vi "点堆模拟机物理参数设置.vi"() -> ()   [LabVIEW 2020]
panel:
  in  "其他说明":string
  in  "文字说明":string
  in  "Lamda 6":sgl
  in  "Lamda 5":sgl
  in  "Lamda 4":sgl
  in  "Lamda 3":sgl
  in  "Lamda 2":sgl
  in  "Beta 6":sgl
  in  "Beta 5":sgl
  in  "Beta 4":sgl
  in  "Beta 3":sgl
  in  "Beta 2":sgl
  in  "取消修改":bool caption="Cancel Button"
  in  "保存修改":bool
  in  "Lamda 1":sgl
  in  "Beta 1":sgl
  in  "源强":sgl
  in  "中子寿命":sgl
  # "点堆模拟机物理参数设置"
  # "（参数对应堆型等）"
  # "（修改日期时间等）"
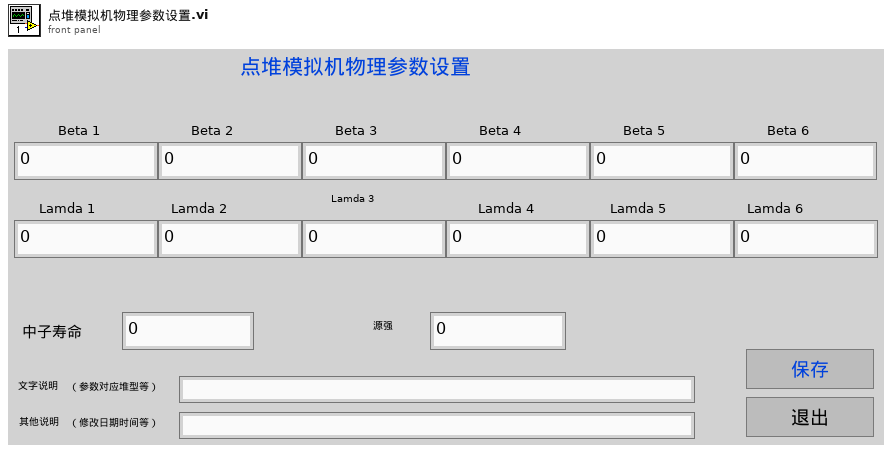
[diagram p1: front panel]
types:
  T1 = enum16{"open", "replace", "create", "open or create", "replace or create", "replace or create with confirmation"}
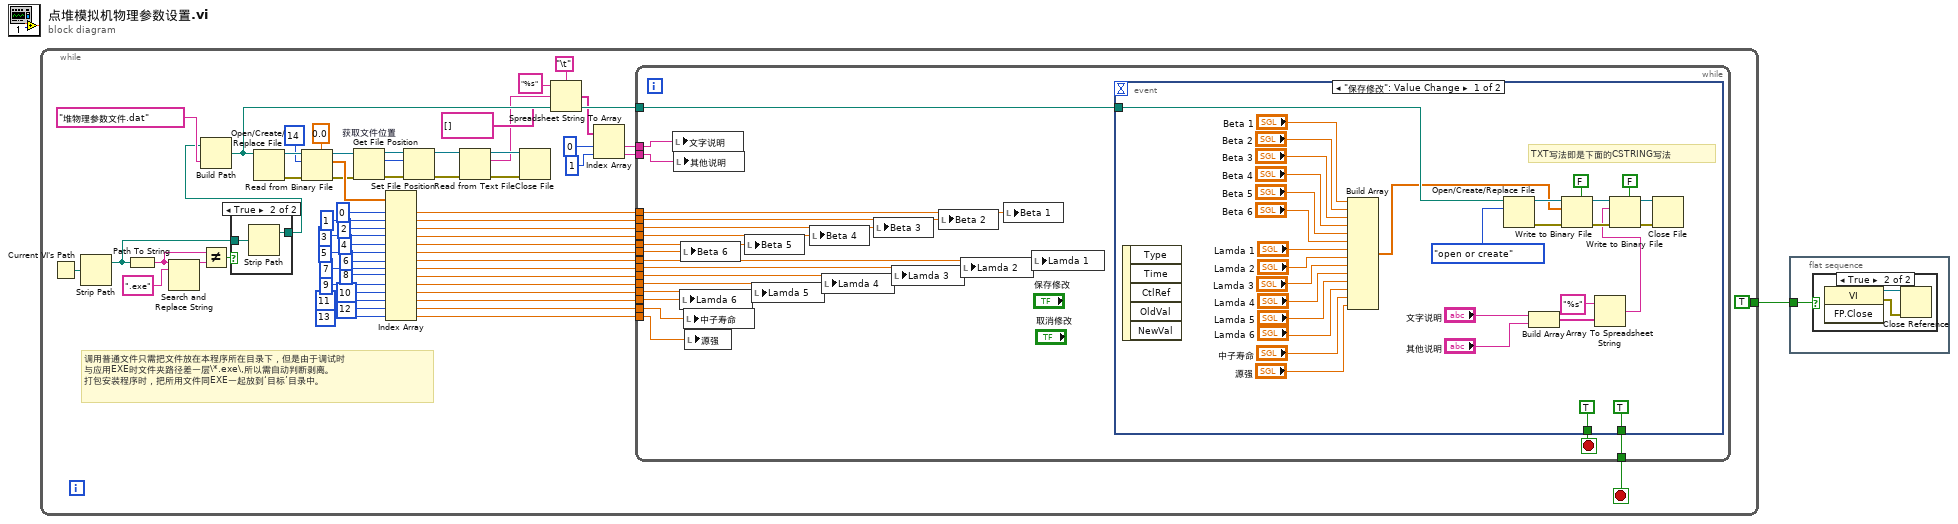
[diagram p0: block diagram]
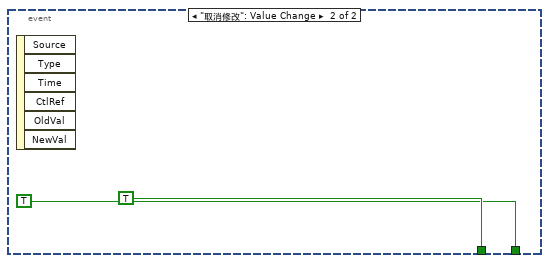
[diagram p4: hidden frame]
diagram:
  n1 = while {
    tunnel: [TRUE] -> w1
    stop <- w38 stop-if-true
    # "调用普通文件只需把文件放在本程序所在目录下，但是由于调试时\n与应用EXE时文件夹路径差一层\\*.exe\\,所以需自动判断剥离。\n打包安装程序时，把所用文件同EXE一起放到‘目标’目录中。"
    n2 = Current VI's Path() -> (path=w9:path)
    n3 = Strip Path(path=w9) -> (stripped path=w4:path)  [unwired: 1 out]
    n4 = Path To String(path=w4) -> (string=w6:string)
    n5 = Search and Replace String(input string=w6, search string=".exe" ("搜索字符串")) -> (result string=w7:string)  [unwired: 6 in, 3 out]
    n6 = Not Equal?(x=w6, y=w7) -> (x != y?=w5:bool)
    n7 = case shown="True" w5 {
      tunnel: w4 -> [w64 w66]
      tunnel: [w64 w65] -> w3
      frame False {
      }
      frame True {
        n8 = Strip Path(path=w66) -> (stripped path=w65:path)  [unwired: 1 out]
      }
    }
    n9 = Build Path(base path=w3, name or relative path="堆物理参数文件.dat") -> (appended path=w36:path)
    n10 = Open/Create/Replace File(file path (use dialog)=w36) -> (refnum out=w49:refnum<file>, error out=w48:errorcluster)  [unwired: 5 in, 1 out]
    n11 = Read from Binary File(5:sgl 0.0 ("byte stream type"), 8:w48, 10:14 ("count"), 11:w49) -> (0:w34:errorcluster, 2:w45:sgl[], 3:w35:refnum<file>)  [unwired: 2 in, 1 out]
    n12 = Get File Position "获取文件位置"(4:w34, 7:w35) -> (0:w43:errorcluster, 2:w19:i64, 3:w44:refnum<file>)
    n13 = Index Array(array=w45, index #1=0, index #2=1, index #3=2, index #4=3, index #5=4, index #6=5, index #7=6, index #8=7, index #9=8, index #10=9, index #11=10, index #12=11, index #13=12, index #14=13) -> (element #1=w33:sgl, element #2=w32:sgl, element #3=w31:sgl, element #4=w30:sgl, element #5=w29:sgl, element #6=w28:sgl, element #7=w27:sgl, element #8=w26:sgl, element #9=w25:sgl, element #10=w24:sgl, element #11=w23:sgl, element #12=w22:sgl, element #13=w21:sgl, element #14=w20:sgl)
    n14 = Set File Position(offset (in bytes) (0)=w19, refnum=w44, error in=w43) -> (refnum out=w18:refnum<file>, error out=w17:errorcluster)  [unwired: 1 in]
    n15 = Read from Text File(file (use dialog)=w18, error in=w17) -> (refnum out=w16:refnum<file>, text=w11:string, error out=w15:errorcluster)  [unwired: 1 in, 2 out]
    n16 = Close File(refnum=w16, error in=w15) -> ()  [unwired: 2 out]
    n17 = Spreadsheet String To Array(delimiter (Tab)="\t", format string="%s", spreadsheet string=w11, array type (2D Dbl)=string[] [] ("添加的数组")) -> (array=w10:string[])
    n18 = Index Array(array=w10, index #1=0 ("index"), index #2=1 ("index")) -> (element #1=w40:string, element #2=w39:string)
    n19 = while {
      tunnel: w33 -> [w85]
      tunnel: w32 -> [w84]
      tunnel: w31 -> [w83]
      tunnel: w30 -> [w82]
      tunnel: w29 -> [w81]
      tunnel: w28 -> [w80]
      tunnel: w27 -> [w79]
      tunnel: w26 -> [w78]
      tunnel: w25 -> [w71]
      tunnel: w24 -> [w77]
      tunnel: w23 -> [w76]
      tunnel: w22 -> [w75]
      tunnel: w36 -> [w73]
      tunnel: w40 -> [w68]
      tunnel: w39 -> [w67]
      tunnel: [w72] -> w38
      tunnel: w21 -> [w70]
      tunnel: w20 -> [w69]
      stop <- w74 stop-if-true
      n20 = local write "文字说明"(w68) -> ()
      n21 = local write "其他说明"(w67) -> ()
      n22 = local write "Lamda 6"(w75) -> ()
      n23 = local write "Beta 6"(w80) -> ()
      n24 = local write "中子寿命"(w70) -> ()
      n25 = local write "源强"(w69) -> ()
      n26 = local write "Beta 5"(w81) -> ()
      n27 = local write "Lamda 5"(w76) -> ()
      n28 = local write "Beta 4"(w82) -> ()
      n29 = local write "Lamda 4"(w77) -> ()
      n30 = local write "Beta 3"(w83) -> ()
      n31 = local write "Lamda 3"(w71) -> ()
      n32 = local write "Beta 2"(w84) -> ()
      n33 = local write "Lamda 2"(w78) -> ()
      n34 = local write "Beta 1"(w85) -> ()
      n35 = local write "Lamda 1"(w79) -> ()
      n36 = event shown="[0] \"保存修改\": Value Change" {
        selector: _ -> [_ _]
        dyn-events: _ -> [_ _]
        timeout: _ -> [_ _]
        tunnel: [TRUE TRUE] -> w74
        tunnel: w73 -> [w107 _]
        tunnel: [TRUE TRUE] -> w72
        event "保存修改": Value Change {
          # "TXT写法即是下面的CSTRING写法"
          n37 = event-data() -> ()  [unwired: 1 in, 5 out]
          n38 = Build Array("Beta 1", "Beta 2", "Beta 3", "Beta 4", "Beta 5", "Beta 6", "Lamda 1", "Lamda 2", "Lamda 3", "Lamda 4", "Lamda 5", "Lamda 6", "中子寿命", "源强") -> (w86:sgl[])
          n39 = Open/Create/Replace File(file path (use dialog)=w107, operation (0:open)=T1."open or create" ("操作(0:open)")) -> (refnum out=w106:refnum<file>, error out=w105:errorcluster)  [unwired: 4 in, 1 out]
          n40 = Build Array("文字说明", "其他说明") -> (w89:string[])
          n41 = Write to Binary File(file (use dialog)=w106, data=w86, error in=w105, 5:FALSE ("预置数组或字符串大小？(T)")) -> (refnum out=w94:refnum<file>, error out=w93:errorcluster)  [unwired: 2 in, 1 out]
          n42 = Array To Spreadsheet String(array=w89, 3:"%s" ("format string")) -> (spreadsheet string=w90:string)  [unwired: 1 in]
          n43 = Write to Binary File(file (use dialog)=w94, data=w90, error in=w93, 5:FALSE ("预置数组或字符串大小？(T)")) -> (refnum out=w96:refnum<file>, error out=w95:errorcluster)  [unwired: 2 in, 1 out]
          n44 = Close File(refnum=w96, error in=w95) -> ()  [unwired: 2 out]
        }
        event "取消修改": Value Change {
          n45 = event-data() -> ()  [unwired: 1 in, 6 out]
        }
      }
    }
  }
  n46 = flat-sequence {
    tunnel: w1 -> [w120]
    frame #0 {
      n47 = case shown="True" w120 {
        frame False {
        }
        frame True {
          n48 = invoke class="VI" method="FP.Close"() -> (reference out=w121:refnum<vi>, error out=w122:errorcluster)  [unwired: 3 in, 1 out]
          n49 = Close Reference(reference=w121, error in (no error)=w122) -> ()  [unwired: 1 out]
        }
      }
    }
  }
